vi "MeasurementInputTest.vi"() -> ()   [LabVIEW 2022 SP3]
uses:
  Meas input Cluster.ctl
  Inst_type.ctl
  portOrDev.ctl
  calType.ctl
  channelState.ctl
panel:
  in  "singleDAQ-port/dev":bool
  in  "singleFs":bool
  in  "Stop":bool
  in  "Clear Solo/Mute":bool
  out "Solo/Mute active":bool
  out "Channel Status Enunciator":string
  in  "scalar":T1 {"Fs" format="%#_pHz"; "syncDelay" format="%#_gms"; "Ch" min=0 step=1}
  in  "NXGarray":T1[](array[typedef])=[{"Type"=enum."Raw voltage", "Label"="sdfasfd", "DAQ"="", "Port"="", "Ch"=0, "Cal"=path "", "calType"=enum."Latest", "Fs"=0.0, "syncDelay"=0.0, "chState"=enum."No Selection"}, {"Type"=enum."Raw voltage", "Label"="Number two", "DAQ"="", "Port"="", "Ch"=4, "Cal"=path "", "calType"=enum."Latest", "Fs"=0.0, "syncDelay"=0.0, "chState"=enum."Mute"}, {"Type"=enum."Raw voltage", "Label"="Hello", "DAQ"="", "Port"="", "Ch"=3, "Cal"=path "", "calType"=enum."Latest", "Fs"=0.0, "syncDelay"=0.0, "chState"=enum."No Selection"}] {"Fs" format="%#_pHz"; "syncDelay" format="%#_gms"; "Ch" min=0 step=1}
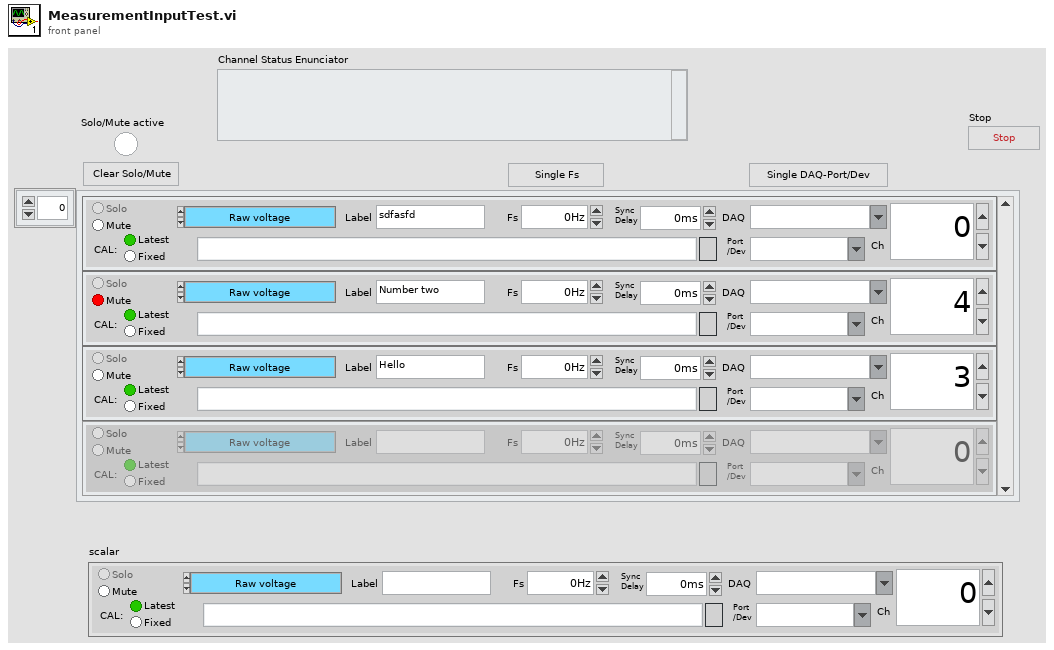
[diagram p1: front panel]
types:
  T1 = typedef "Meas input Cluster.ctl" = cluster{"Type":T2, "Label":string, "DAQ":string, "Port":T3, "Ch":i32, "Cal":path, "calType":T4, "Fs":dbl, "syncDelay":dbl, "chState":T5}
  T2 = typedef "Inst_type.ctl" = enum16{"Raw voltage", "Raw with zero offsetting", "Propeller anemometer", "Pressure Transducer", "Pitot-static tube", "Hot wire", "Cross wire 1", "Cross wire 2", "Generic Linear", "Generic Polynomial", "Generic BackPoly", "Fast FID", "Thermocouple", "Cold wire", "Pulsed Wire", "LDA Vel", "LDA Tran time", "LDA Arr time", "Microphone"}
  T3 = typedef "portOrDev.ctl" = string
  T4 = typedef "calType.ctl" = enum32{"Latest", "Fixed"}
  T5 = typedef "channelState.ctl" = enum32{"No Selection", "Solo", "Mute"}
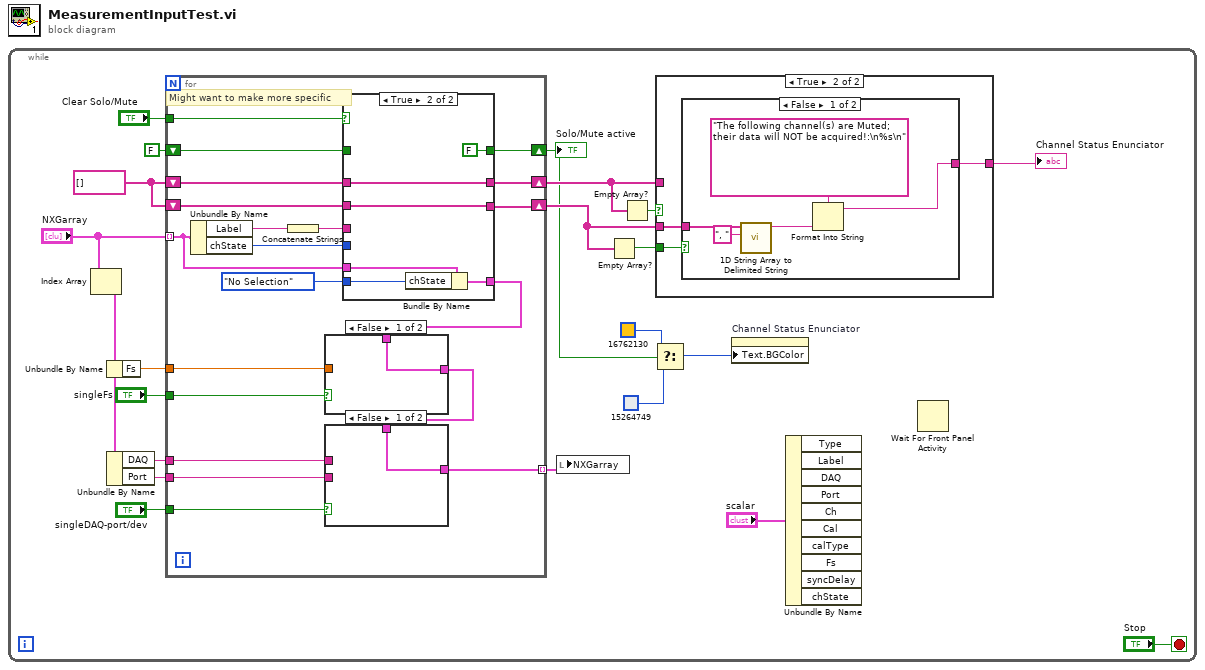
[diagram p0: block diagram]
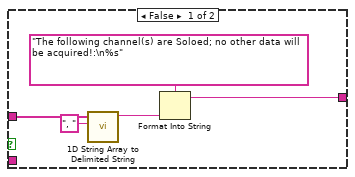
[diagram p2: hidden frame]
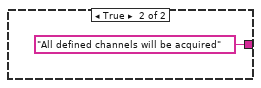
[diagram p3: hidden frame]
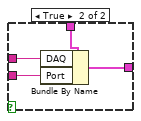
[diagram p4: hidden frame]
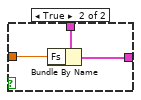
[diagram p5: hidden frame]
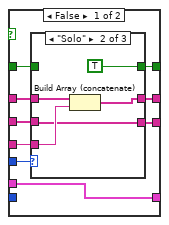
[diagram p6: hidden frame]
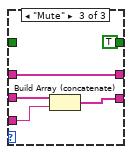
[diagram p8: hidden frame]
diagram:
  n1 = while {
    stop <- "Stop" stop-if-true
    w22 = string[] []
    n2 = Index Array(array="NXGarray") -> (element=w5:T1)  [unwired: 1 in]
    n3 = Unbundle By Name(w5) -> ("Fs"=w8:dbl)
    n4 = Unbundle By Name(w5) -> ("DAQ"=w4:string, "Port"=w3:T3)
    n5 = for {
      tunnel: "NXGarray" -> [w45] mode=indexing
      shift-right: [w54] -> w21
      shift-left: w22 -> [w55]
      shift-right: [w51] -> w18
      shift-left: w22 -> [w52]
      shift-right: [w49] -> w9
      shift-left: FALSE -> [w48]
      tunnel: "Clear Solo/Mute" -> [w47]
      tunnel: w8 -> [w44]
      tunnel: "singleFs" -> [w42]
      tunnel: w4 -> [w40]
      tunnel: w3 -> [w39]
      tunnel: "singleDAQ-port/dev" -> [w38]
      tunnel: [w37] -> w1 mode=indexing
      # "Might want to make more specific"
      n6 = Unbundle By Name(w45) -> ("Label"=w53:string, "chState"=w56:T5)
      n7 = Concatenate Strings(w53) -> (w50:string)
      n8 = case shown="True" w47 {
        tunnel: w56 -> [w74 _]
        tunnel: w55 -> [w73 w89]
        tunnel: [w72 w89] -> w54
        tunnel: w52 -> [w71 w88]
        tunnel: [w70 w88] -> w51
        tunnel: w50 -> [w69 _]
        tunnel: [w68 FALSE] -> w49
        tunnel: w48 -> [w67 _]
        tunnel: w45 -> [w66 w92]
        tunnel: channelState."No Selection" ("chState") -> [_ w91]
        tunnel: [w66 w90] -> w43
        frame False {
          n9 = case shown="\"Solo\"" w74 {
            tunnel: w73 -> [w77 w82 w85]
            tunnel: [w77 w80 w85] -> w72
            tunnel: w69 -> [_ w81 w84]
            tunnel: w71 -> [w76 w79 w87]
            tunnel: [w76 w79 w86] -> w70
            tunnel: [w75 TRUE TRUE] -> w68
            tunnel: w67 -> [w75 _ _]
            frame "No Selection", Default {
            }
            frame "Solo" {
              n10 = Build Array (concatenate)(w82, w81) -> (w80:string[])
            }
            frame "Mute" {
              n11 = Build Array (concatenate)(w87, w84) -> (w86:string[])
            }
          }
        }
        frame True {
          n12 = Bundle By Name(cluster=w92, "chState"=w91) -> (w90:T1)
        }
      }
      n13 = case shown="False" w42 {
        tunnel: w44 -> [_ w65]
        tunnel: w43 -> [w62 w64]
        tunnel: [w62 w63] -> w41
        frame False {
        }
        frame True {
          n14 = Bundle By Name(cluster=w64, "Fs"=w65) -> (w63:T1)
        }
      }
      n15 = case shown="False" w38 {
        tunnel: w41 -> [w57 w61]
        tunnel: w40 -> [_ w60]
        tunnel: w39 -> [_ w59]
        tunnel: [w57 w58] -> w37
        frame False {
        }
        frame True {
          n16 = Bundle By Name(cluster=w61, "DAQ"=w60, "Port"=w59) -> (w58:T1)
        }
      }
    }
    "Solo/Mute active" <- w9
    n17 = local write "NXGarray"(w1) -> ()
    n18 = Empty Array?(array=w18) -> (empty?=w17:bool)
    n19 = Empty Array?(array=w21) -> (empty?=w19:bool)
    n20 = Select(t=u32 16762130 ("Text.Colors:BG Color"), s=w9, f=u32 15264749 ("Text.Colors:BG Color")) -> (s? t:f=w12:u32)
    n21 = case shown="True" w19 {
      tunnel: w21 -> [w26 _]
      tunnel: [w23 w28] -> w20
      tunnel: w18 -> [_ w30]
      tunnel: w17 -> [_ w29]
      frame False {
        n22 = call <vilib>:"1D String Array to Delimited String.vi"("delimiter"=", ", "string array"=w26) -> ("delimited string"=w24:string)  [unwired: 9 in]
        n23 = Format Into String(format string="The following channel(s) are Soloed; no other data will be acquired!:\n%s", w24) -> (resulting string=w23:string)  [unwired: 2 in, 1 out]
      }
      frame True {
        n24 = case shown="False" w29 {
          tunnel: w30 -> [w34 _]
          tunnel: [w31 "All defined channels will be acquired"] -> w28
          frame False {
            n25 = call <vilib>:"1D String Array to Delimited String.vi"("delimiter"=", ", "string array"=w34) -> ("delimited string"=w33:string)  [unwired: 9 in]
            n26 = Format Into String(format string="The following channel(s) are Muted; their data will NOT be acquired!:\n%s\n", w33) -> (resulting string=w31:string)  [unwired: 2 in, 1 out]
          }
          frame True {
          }
        }
      }
    }
    "Channel Status Enunciator" <- w20
    n27 = property on="Channel Status Enunciator" class="Str"("Text.BGColor"=w12) -> ()  [unwired: 2 in, 2 out]
    n28 = Unbundle By Name("scalar") -> ()  [unwired: 10 out]
    n29 = Wait For Front Panel Activity() -> ()  [unwired: 3 in, 1 out]
  }
